vi "Mouse Up.vi"(7 "Map Model in":refnum<class "Map Model.lvclass">, 8 "error in (no error)":errorcluster, 10 "Position":T1, 11 "Undoable Tool in":refnum<class "Undoable Tool.lvclass">) -> (0 "error out":errorcluster, 3 "Undoable Tool out":refnum<class "Undoable Tool.lvclass">, 5 "Map Model out":refnum<class "Map Model.lvclass">)   [LabVIEW 2020, in "Map Model.lvlib" / "Undoable Tool.lvclass"]
uses:
  Undoable Tool.lvclass
  E:/Project/Labview-Projects/Completed projects/Map Editor/Models/Map Model/Tools/Tool/Tool.lvclass
  <vilib>/Utility/miscctls.llb/LVPoint32TypeDef.ctl
  Map Model/Map Model.lvclass
  Tool/Tool.lvclass/Tool.ctl
  Map Model/Map Model.lvclass/Map Model.ctl
  Undoable Tool.lvclass/Undoable Tool.ctl
  Tool/Tool.lvclass
  Stack/Stack.lvclass
panel:
  # "NOTICE -- YOU MUST LEAVE THIS NOTICE IN PLACE.\n\nCopyright (c) 2017, LIANG LIU Shawn.Liu.cn@gmail.com\nAll rights reserved.\n\nRedistribution and use in source and binary forms, with or without modification, are permitted provided that the following conditions are met:\n-Redistributions of source code must retain the above copyright notice, this list of conditions and the following disclaimer.\n-Redistributions in binary form must reproduce the above copyright notice, this list of conditions and the following disclaimer in the documentation and/or other materials provided with the distribution.\n-Neither the name of the eLp nor the names of its contributors may be used to endorse or promote products derived from this software without specific prior written permission.\n\nTHIS SOFTWARE IS PROVIDED BY THE COPYRIGHT HOLDERS AND CONTRIBUTORS \"AS IS\" AND ANY EXPRESS OR IMPLIED WARRANTIES, INCLUDING, BUT NOT LIMITED TO, THE IMPLIED WARRANTIES OF MERCHANTABILITY AND FITNESS FOR A PARTICULAR PURPOSE ARE DISCLAIMED. IN NO EVENT SHALL THE COPYRIGHT HOLDER OR CONTRIBUTORS BE LIABLE FOR ANY DIRECT, INDIRECT, INCIDENTAL, SPECIAL, EXEMPLARY, OR CONSEQUENTIAL DAMAGES (INCLUDING, BUT NOT LIMITED TO, PROCUREMENT OF SUBSTITUTE GOODS OR SERVICES; LOSS OF USE, DATA, OR PROFITS; OR BUSINESS INTERRUPTION) HOWEVER CAUSED AND ON ANY THEORY OF LIABILITY, WHETHER IN CONTRACT, STRICT LIABILITY, OR TORT (INCLUDING NEGLIGENCE OR OTHERWISE) ARISING IN ANY WAY OUT OF THE USE OF THIS SOFTWARE, EVEN IF ADVISED OF THE POSSIBILITY OF SUCH DAMAGE."
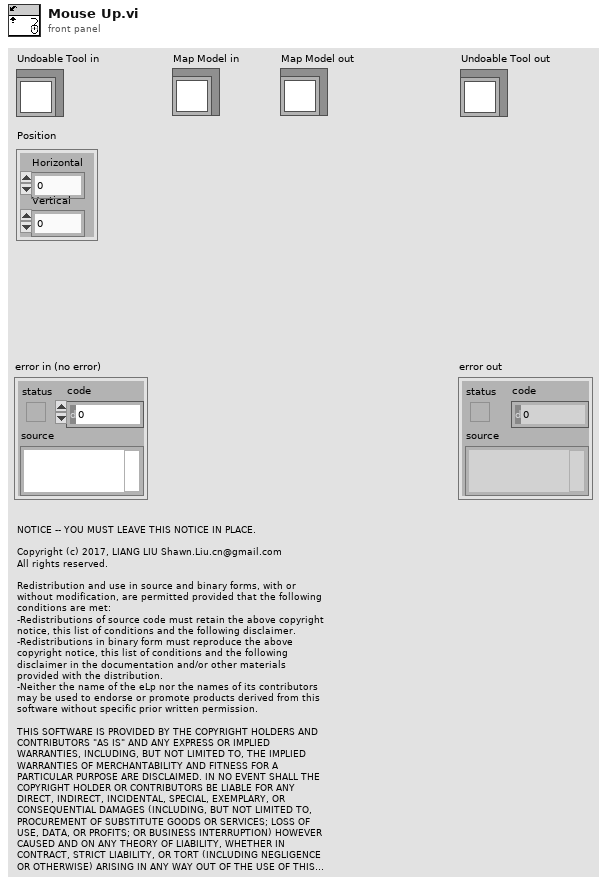
[diagram p1: front panel]
types:
  T1 = typedef "LVPoint32TypeDef.ctl" = cluster{"Horizontal":i32, "Vertical":i32}
  T2 = enum8{"Enabled", "Disabled", "Disabled and Grayed Out"}
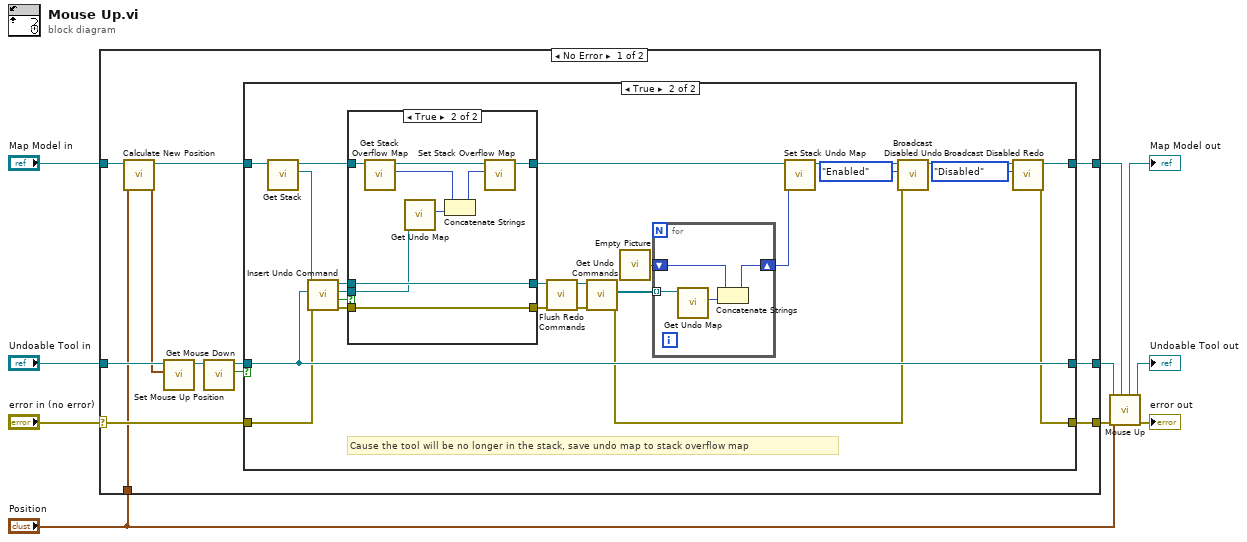
[diagram p0: block diagram]
diagram:
  n1 = case shown="No Error" "error in (no error)" {
    selector: "error in (no error)" -> [w19 w68]
    tunnel: "Map Model in" -> [w22 w67]
    tunnel: "Undoable Tool in" -> [w21 w66]
    tunnel: [w20 w68] -> w6
    tunnel: [w18 w66] -> w4
    tunnel: [w17 w67] -> w3
    tunnel: "Position" -> [w16 _]
    frame No Error {
      n2 = call "Calculate New Position.vi"("Position in"=w16, "Map Model in"=w22) -> ("Position out"=w11:T1, "Map Model out"=w12:refnum<class "Map Model.lvclass">)  [unwired: 8 in]
      n3 = call "Set Mouse Up Position.vi"("Mouse Up Position"=w11, "Tool in"=w21) -> ("Tool out"=w13:refnum<class "Undoable Tool.lvclass">)  [unwired: 9 in]
      n4 = call "Get Mouse Down.vi"("Tool in"=w13) -> ("Mouse Down"=w14:bool, "Tool out"=w15:refnum<class "Undoable Tool.lvclass">)  [unwired: 9 in]
      n5 = case shown="True" w14 {
        tunnel: w12 -> [w24 w49]
        tunnel: [w25 w28] -> w20
        tunnel: [w24 w37] -> w17
        tunnel: w15 -> [w23 w40]
        tunnel: w19 -> [w25 w27]
        tunnel: [w23 w40] -> w18
        frame False {
        }
        frame True {
          # "Cause the tool will be no longer in the stack, save undo map to stack overflow map"
          n6 = call "Get Stack.vi"("Map Model in"=w49) -> ("Stack"=w43:refnum<class "Stack.lvclass">, "Map Model out"=w47:refnum<class "Map Model.lvclass">)  [unwired: 9 in]
          n7 = call "Insert Undo Command.vi"("error in (no error)"=w27, "Undo Command"=w40, "Stack in"=w43) -> ("error out"=w41:errorcluster, "Overflow"=w44:bool, "Overflow Undo Command"=w45:refnum<class "Undoable Tool.lvclass">, "Stack out"=w46:refnum<class "Stack.lvclass">)  [unwired: 5 in]
          n8 = case shown="True" w44 {
            tunnel: w46 -> [w56 w65]
            tunnel: w45 -> [_ w61]
            tunnel: [w56 w65] -> w39
            tunnel: w47 -> [w55 w64]
            tunnel: [w55 w62] -> w32
            tunnel: w41 -> [w54 w57]
            tunnel: [w54 w57] -> w38
            frame False {
            }
            frame True {
              n9 = call "Get Stack Overflow Map.vi"("Map Model in"=w64) -> ("Stack Overflow Map"=w59:picture, "Map Model out"=w63:refnum<class "Map Model.lvclass">)  [unwired: 9 in]
              n10 = call "Get Undo Map.vi"("Undoable Tool in"=w61) -> ("Undo Map"=w60:picture)  [unwired: 9 in, 1 out]
              n11 = Concatenate Strings(w59, w60) -> (w58:picture)
              n12 = call "Set Stack Overflow Map.vi"("Stack Overflow Map"=w58, "Map Model in"=w63) -> ("Map Model out"=w62:refnum<class "Map Model.lvclass">)  [unwired: 9 in]
            }
          }
          n13 = call "Flush Redo Commands.vi"("error in (no error)"=w38, "Stack in"=w39) -> ("error out"=w29:errorcluster, "Stack out"=w30:refnum<class "Stack.lvclass">)  [unwired: 8 in]
          n14 = call "Get Undo Commands.vi"("error in (no error)"=w29, "Stack in"=w30) -> ("error out"=w26:errorcluster, "Undo Commands"=w33:refnum<class "Undoable Tool.lvclass">[])  [unwired: 7 in, 1 out]
          n15 = call "Empty Picture"() -> ("empty picture"=w35:picture)
          n16 = for {
            tunnel: w33 -> [w53] mode=indexing
            shift-right: [w50] -> w34
            shift-left: w35 -> [w51]
            n17 = call "Get Undo Map.vi"("Undoable Tool in"=w53) -> ("Undo Map"=w52:picture)  [unwired: 9 in, 1 out]
            n18 = Concatenate Strings(w51, w52) -> (w50:picture)
          }
          n19 = call "Set Stack Undo Map.vi"("Stack Undo Map"=w34, "Map Model in"=w32) -> ("Map Model out"=w31:refnum<class "Map Model.lvclass">)  [unwired: 9 in]
          n20 = call "Broadcast Disabled Undo.vi"("error in (no error)"=w26, "Disabled Undo"=T2."Enabled", "Map Model in"=w31) -> ("Map Model out"=w48:refnum<class "Map Model.lvclass">)  [unwired: 7 in, 1 out]
          n21 = call "Broadcast Disabled Redo.vi"("Disabled Redo"=T2."Disabled", "Map Model in"=w48) -> ("error out"=w28:errorcluster, "Map Model out"=w37:refnum<class "Map Model.lvclass">)  [unwired: 8 in]
        }
      }
    }
    frame Error {
    }
  }
  n22 = call-parent "Mouse Up.vi"("Map Model in"=w3, "error in (no error)"=w6, "Position"="Position", "Tool in"=w4) -> ("error out"=→"error out":errorcluster, "Tool out"=→"Undoable Tool out":refnum<class "Undoable Tool.lvclass">, "Map Model out"=→"Map Model out":refnum<class "Map Model.lvclass">)  [unwired: 5 in]
